vi "Get NamedUnbundler.vi"(8 "error in (no error)":errorcluster, 10 "Label":string, 11 "Owner VI in":refnum<vi>) -> (0 "error out":errorcluster, 1 "Found ?":bool, 2 "NamedUnbundler ref out":refnum<vi>, 3 "Owner VI out":refnum<vi>)   [LabVIEW 2019, in "gRPC Scripting Tools.lvlib"]
uses:
  gRPC Scripting Tools.lvlib
  <vilib>/Utility/traverseref.llb/TRef TravTarget.ctl
  <vilib>/Utility/traverseref.llb/VI Scripting - Traverse.lvlib
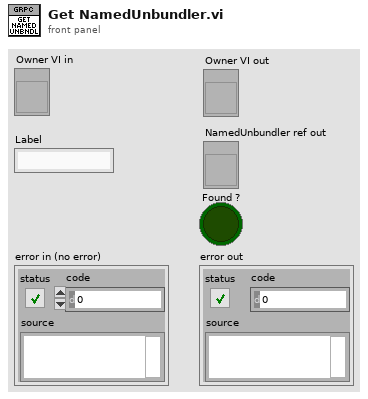
[diagram p1: front panel]
types:
  T1 = typedef "TRef TravTarget.ctl" = enum16{"FP", "BD", "Other"}
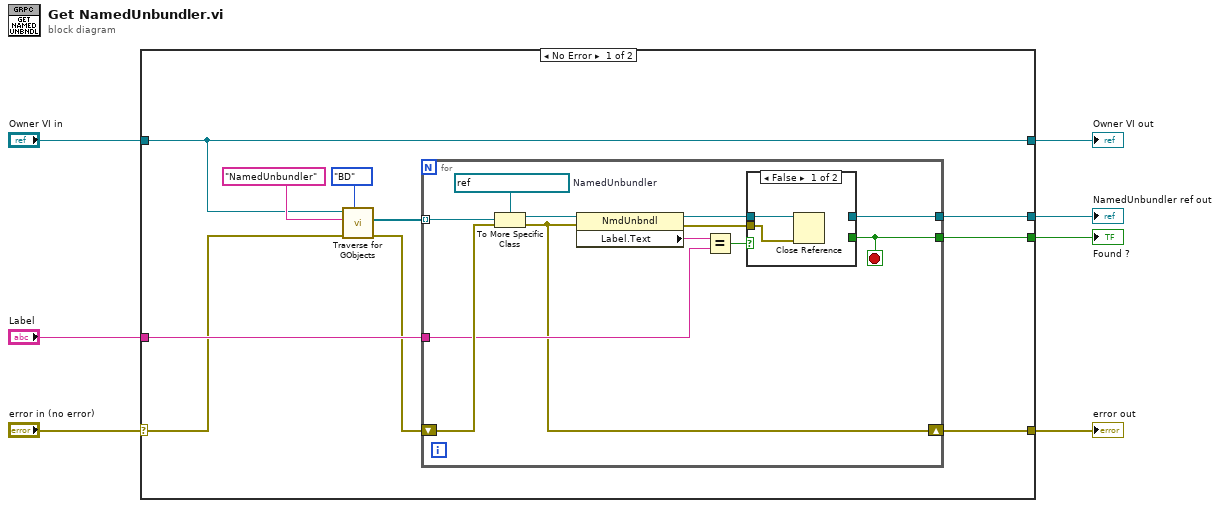
[diagram p0: block diagram]
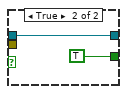
[diagram p2: hidden frame]
diagram:
  n1 = case shown="No Error" "error in (no error)" {
    selector: "error in (no error)" -> [w11 w34]
    tunnel: "Label" -> [w17 _]
    tunnel: "Owner VI in" -> [w10 w35]
    tunnel: [w8 w34] -> w5
    tunnel: [w12 _] -> w1
    tunnel: [w10 w35] -> w3
    tunnel: [w9 _] -> w2
    frame No Error {
      n2 = call <vilib>:"Traverse for GObjects.vi"("Traverse Target"=TRef_TravTarget."BD", "error in (no error)"=w11, "Class Name"="NamedUnbundler", "VI Refnum"=w10) -> ("error out"=w13:errorcluster, "References"=w16:refnum<vi>[])  [unwired: 4 in, 2 out]
      n3 = for {
        tunnel: w16 -> [w29] mode=indexing
        tunnel: w17 -> [w24]
        tunnel: [w21] -> w12
        tunnel: [w19] -> w9
        shift-right: [w18] -> w8
        shift-left: w13 -> [w27]
        stop <- w19 stop-if-true
        w28 = refnum<vi> refnum  # NamedUnbundler
        n4 = To More Specific Class(target class=w28, reference=w29, error in=w27) -> (specific class reference=w26:refnum<vi>, error out=w18:errorcluster)
        n5 = property class="NmdUnbndl"(reference=w26, error in=w18) -> (reference out=w22:refnum<vi>, error out=w20:errorcluster, "Label.Text"=w25:string)
        n6 = Equal?(x=w25, y=w24) -> (x = y?=w23:bool)
        n7 = case shown="False" w23 {
          tunnel: w22 -> [w31 w33]
          tunnel: [_ w33] -> w21
          tunnel: [_ TRUE] -> w19
          tunnel: w20 -> [w30 _]
          frame False {
            n8 = Close Reference(reference=w31, error in (no error)=w30) -> ()  [unwired: 1 out]
          }
          frame True {
          }
        }
      }
    }
    frame Error {
    }
  }
  "error out" <- w5
  "Owner VI out" <- w3
  "Found ?" <- w2
  "NamedUnbundler ref out" <- w1
